vi "linear interpolation.vi"(5 "dx":fxp<+/-,32,32>, 6 "dy":fxp<+/-,52,52>, 7 "y":fxp<+/-,19,19>) -> (3 "predicted y":fxp<+/-,24,24>)   [LabVIEW 2011, in "EPS_Timekeeper.lvlib"]
uses:
  <vilib>/rvi/FXPMathLib/FxpDiv/subVIs/nifxpmath_Div_SimConfig.ctl
  <vilib>/rvi/FXPMathLib/FxpDiv/simVIs/DllFxpDivTemp_sub.vi
  <vilib>/rvi/FXPMathLib/FxpDiv/XNode/nifxpmath_Div.xnode
  <vilib>/addons/Electrical Power/Example Support/PMU/Time Keeper/EPS_Timekeeper.lvlib
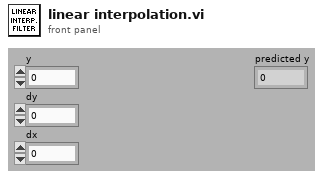
[diagram p1: front panel]
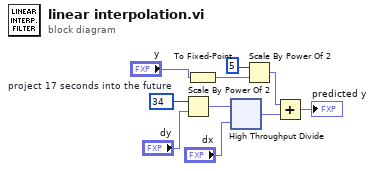
[diagram p0: block diagram]
diagram:
  w9 = 34  # project 17 seconds into the future
  n1 = Scale By Power Of 2(n=w9, x="dy") -> (x*2^n=w7:fxp<+/-,52,52>)
  n2 = To Fixed-Point(number="y") -> (fixed-point=w1:fxp<+/-,24,24>)  [unwired: 1 in]
  n3 = xnode "High Throughput Divide"("x"=w7, "y"="dx") -> ("x/y"=w5:fxp<+/-,52,52>)
  n4 = Scale By Power Of 2(n=5, x=w1) -> (x*2^n=w3:fxp<+/-,24,24>)
  n5 = Add(x=w3, y=w5) -> (x+y=→"predicted y":fxp<+/-,24,24>)
